vi "Update_Reg_Tracker w_Fuses Readback.vi"(8 "Error In":errorcluster, 10 "Master_Register_Data_Array_In":T1 {"Address" format="%.0x"}, 11 "Readback_Array":T2[](array[typedef]) {"Address" format="%.0x"}) -> (0 "Error Out":errorcluster, 3 "Master_Register_Data_Array_Out":T1 {"Address" format="%.0x"})   [LabVIEW 2013]
uses:
  Controls/Reg_Address_Data.ctl
  Controls/Master_Reg_Data_Array.ctl
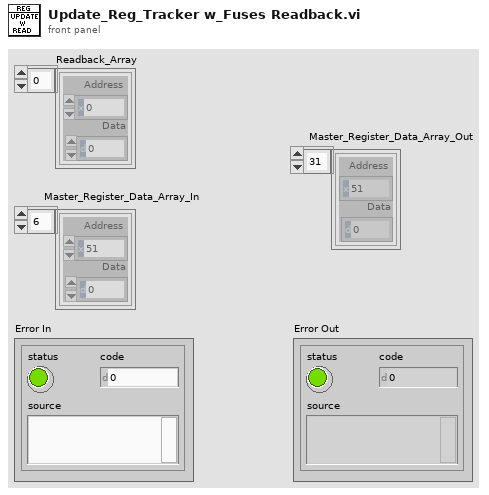
[diagram p1: front panel]
types:
  T1 = typedef "Master_Reg_Data_Array.ctl" = T2[]
  T2 = typedef "Reg_Address_Data.ctl" = cluster{"Address":u8, "Data":u8}
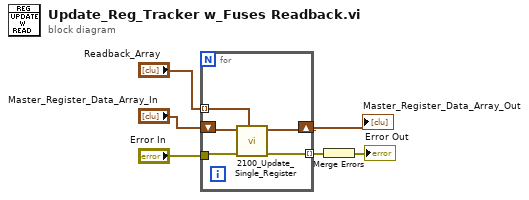
[diagram p0: block diagram]
diagram:
  n1 = for {
    tunnel: "Readback_Array" -> [w10] mode=indexing
    tunnel: [w9] -> w3 mode=indexing
    tunnel: "Error In" -> [w8]
    shift-right: [w7] -> w1
    shift-left: "Master_Register_Data_Array_In" -> [w11]
    n2 = call "2100_Update_Single_Register.vi"("Reg_Address_Data"=w10, "Error In"=w8, "Master_Register_Data_Array_In"=w11) -> ("Error Out"=w9:errorcluster, "Master_Register_Data_Array_Out"=w7:T1)  [unwired: 6 in, 1 out]
  }
  "Master_Register_Data_Array_Out" <- w1
  n3 = Merge Errors(w3) -> (→"Error Out":errorcluster)
